vi "LVFPGA Tx.vi"(0 "device name":string="RIO0", 1 "Enabled Channels":string(combo)="0", 5 "IQ rate":dbl=10000000.0 caption="IQ Rate" format="%#.3pS/s", 7 "number of samples":i64=16384 caption="Number of Samples", 9 "run duration":dbl=5.0 format="%#_13g", 11 "error in":errorcluster) -> (6 "coerced IQ rate":dbl format="%#_6p", 8 "underflow":bool, 10 "overflow":bool, 15 "error out":errorcluster)   [LabVIEW 2015]
doc: "This template is for the Simple NI-USRP Streaming design, a design that shows the basics of streaming data to an NI USRP-294x/295x device. Refer to the block diagram for more information about how to use this template."
uses:
  SubVIs/niusrprios Write Tx Data (I16 multi).vi
  SubVIs/niusrprios Start Trigger.ctl
  SubVIs/niusrprios Configure Signal (Level).vi
  SubVIs/niusrprios Generate Waveform (Interleaved).vi
panel:
  in  "which bitfile":string(combo)="Time"
  in  "Reference Frequency Source":string(combo)="Internal"
  out "generating":bool caption="Generating"
  in  "number of samples is finite":bool
  in  "stop":bool
  # "Tx Streaming"
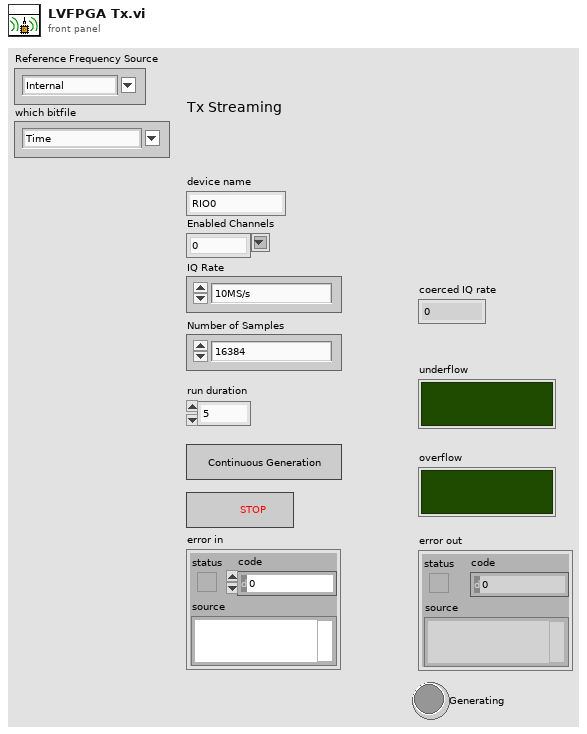
[diagram p1: front panel]
types:
  T1 = typedef "niusrprios Start Trigger.ctl" = enum8{"Software", "Digital Edge", "Rx Start Trigger", "Tx Start Trigger", "Immediate", "Future Time Event"}
  T2 = cluster{"antenna":string, "frequency":dbl, "lo frequency":dbl, "level":dbl}
  T3 = cluster{"channel enable":bool, "channel configuration":cluster{"antenna":string, "frequency":dbl, "lo frequency":dbl, "level":dbl}}
  T4 = cluster{"antenna":string, "frequency":dbl, "lo frequency":dbl, "level":dbl}[]
  T5 = typedef "niUsrpRio Config v1 Host.lvlib/niUsrpRio Session.ctl" = cluster{"FPGA Interface":refnum<k20>, "RIO Interface Number":u32, "Data Clock Rate":u32, "FPGA Data Clock Rate":u32, "Global Settings Register Bus":T6, "Radio 0 Settings Register Bus":T6, "Radio 1 Settings Register Bus":T6, "Radio Settings Bus Semaphore":T7, "DB Queues":T8[], "Characterization Data Valid?":bool, "EEPROM Header":T9, "Device Data Header":T10, "EEPROM Characterization Header":T11, "Characterization Data":T12[], "FPGA Current Version":u32, "FPGA Oldest Compatible Version":u32, "Fixed Logic Current Version":u32, "Fixed Logic Oldest Compatible Version":u32, "FPGA Radio Settings Bus Current Version":u32, "FPGA Radio Settings Bus Oldest Compatible Version":u32, "FPGA Board Config Current Version":u32, "FPGA Board Config Oldest Compatible Version":u32, "Daughterboard Clock Rate":u32}
  T6 = typedef "niInstr Register Bus v0 Host.lvlib/Register Bus Session.ctl" = refnum<queue>
  T7 = typedef "Semaphore RefNum" = refnum<k1>
  T8 = typedef "niUsrpRio Config v1 Host.lvlib/DB Queue Reference.ctl" = refnum<queue>
  T9 = typedef "niUsrpRio Config v1 Host.lvlib/EEPROM Header.ctl" = cluster{"Checksum":u32, "Product Code":u16, "Hardware Current Version":u16, "Hardware Oldest Compatible Version":u16, "EEPROM Map Current Version":u16, "EEPROM Map Oldest Compatible Version":u16, "User Password":string, "Pointer to Factory Header":u32, "Pointer to User Header":u32, "Recommended Interval":u16, "Number of Reserved Bytes":i32, "Number of Daughterboards":u8, "Daughterboard IDs":u16[], "Daughterboard Serial Numbers":string[]}
  T10 = typedef "niUsrpRio Config v1 Host.lvlib/EEPROM Device Data Header.ctl" = cluster{"Checksum":u32, "Number of Channels":u8, "Number of Gain Settings":u16[], "Pointer to Characterization Data":u32[], "Number of Reserved Bytes":i32, "Number of Frequencies":u16[]}
  T11 = typedef "niUsrpRio Config v1 Host.lvlib/EEPROM Characterization Header.ctl" = cluster{"Checksum":u32, "Date":timestamp, "Temperature":sgl, "Misc. Info":string, "Pointer to Device Data Header":u32, "Number of Reserved Bytes":i32}
  T12 = typedef "niUsrpRio Config v1 Host.lvlib/Characterization Data.ctl" = cluster{"Gains[dB]":dbl[], "Frequencies [Hz]":dbl[], "IQ Imbalance Table":T13[], "Measured Gains[dB]":dbl[][]}
  T13 = typedef "niUsrpRio Config v1 Host.lvlib/IQ Imbalance.ctl" = cluster{"Gain Imbalance [linear]":dbl, "Phase Imbalance [radians]":dbl, "Offset":cdb}
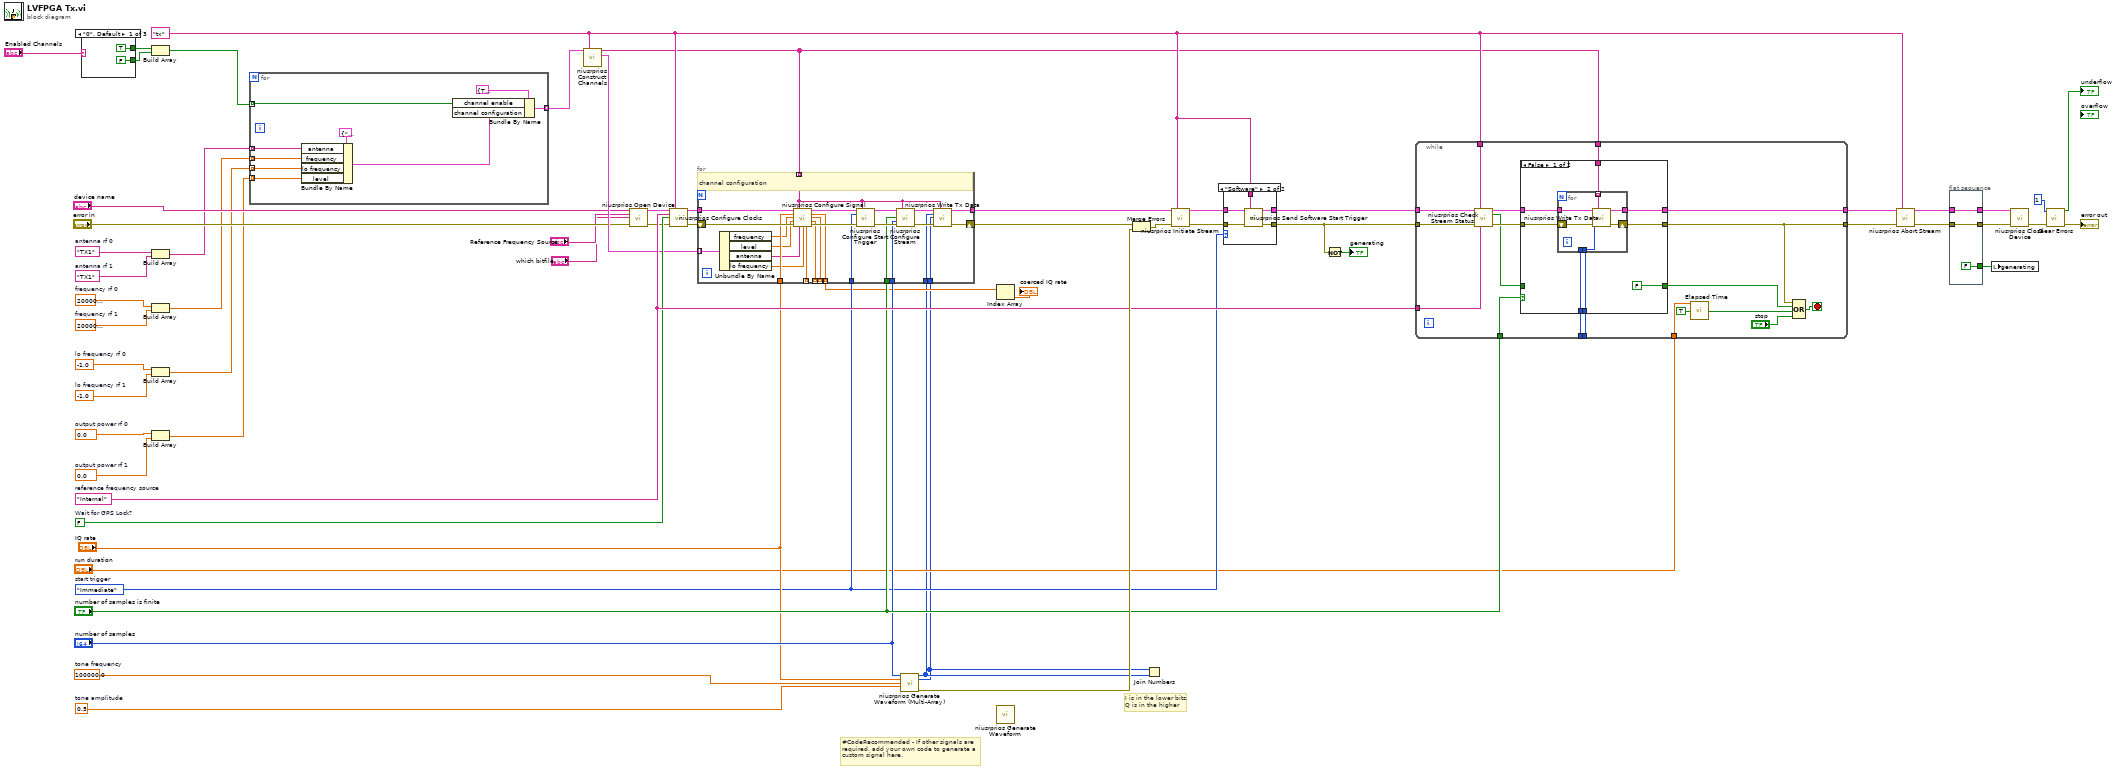
[diagram p0: block diagram]
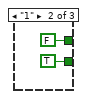
[diagram p2: hidden frame]
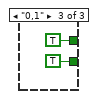
[diagram p3: hidden frame]
diagram:
  w48 = 100000.0  # tone frequency
  w39 = niusrprios_Start_Trigger."Immediate"  # start trigger
  w62 = "Internal"  # reference frequency source
  w53 = 0.0  # output power rf 1
  w52 = 0.0  # output power rf 0
  w54 = -1.0  # lo frequency rf 1
  w55 = -1.0  # lo frequency rf 0
  w56 = 2000000000.0  # frequency rf 1
  w57 = 2000000000.0  # frequency rf 0
  w59 = "TX1"  # antenna rf 1
  w58 = "TX1"  # antenna rf 0
  w40 = FALSE  # Wait for GPS Lock?
  w47 = 0.5  # tone amplitude
  w35 = "tx" ("scope")
  # "I is in the lower bits,\nQ is in the higher"
  # "#CodeRecommended - If other signals are required, add your own code to generate a custom signal here."
  n1 = case shown="\"0\", Default" "Enabled Channels" {
    tunnel: [TRUE FALSE TRUE] -> w21
    tunnel: [FALSE TRUE TRUE] -> w20
    frame "0", Default {
    }
    frame "1" {
    }
    frame "0,1" {
    }
  }
  n2 = Build Array(w21, w20) -> (w12:bool[])
  n3 = Build Array(w58, w59) -> (w11:string[])
  n4 = Build Array(w57, w56) -> (w10:dbl[])
  n5 = Build Array(w55, w54) -> (w9:dbl[])
  n6 = Build Array(w52, w53) -> (w8:dbl[])
  n7 = for {
    tunnel: w12 -> [w77] mode=indexing
    tunnel: w11 -> [w75] mode=indexing
    tunnel: w10 -> [w74] mode=indexing
    tunnel: w9 -> [w73] mode=indexing
    tunnel: w8 -> [w72] mode=indexing
    tunnel: [w70] -> w7 mode=indexing
    n8 = Bundle By Name(cluster=T2 {"antenna"="", "frequency"=0.0, "lo frequency"=0.0, "level"=0.0} ("channel configuration"), "antenna"=w75, "frequency"=w74, "lo frequency"=w73, "level"=w72) -> (w71:T2)
    n9 = Bundle By Name(cluster=T3 {"channel enable"=TRUE, "channel configuration"={"antenna"="RX1", "frequency"=2000000000.0, "lo frequency"=-1.0, "level"=0.0}} ("channel configuration"), "channel enable"=w77, "channel configuration"=w71) -> (w70:T3)
  }
  n10 = call "niusrprios Construct Channels.vi"("channel configurations"=w7, "scope"=w35) -> ("enabled channels"=w34:string[], "enabled channel configurations"=w33:T4)  [unwired: 12 in]
  n11 = call "niusrprios Open Device.vi"("USRP RIO device"="device name", "Reference Frequency Source"="Reference Frequency Source", "which bitfile"="which bitfile", "error in"="error in") -> ("niUsrpRio Session (out)"=w32:T5, "error out"=w31:errorcluster)  [unwired: 10 in]
  n12 = call "niusrprios Configure Clocks.vi"("niUsrpRio Session"=w32, "scope"=w35, "Reference Frequency Source"=w62, "GPSDO Power Enable"=w40, "error in"=w31) -> ("niUsrpRio Session (out)"=w29:T5, "error out"=w30:errorcluster)  [unwired: 9 in]
  n13 = call "niusrprios Generate Waveform (Multi-Array).vi"("number of samples"="number of samples", "sample rate"="IQ rate", "tone frequency"=w48, "amplitude"=w47) -> ("I"=w4:i16[], "Q"=w3:i16[], "error out"=w63:errorcluster)  [unwired: 8 in, 1 out]
  n14 = for {
    tunnel: [w87] -> _ mode=indexing
    tunnel: [w92] -> w27
    tunnel: w39 -> [w102]
    tunnel: "number of samples" -> [w97]
    tunnel: "number of samples is finite" -> [w96]
    shift-right: [w94] -> w26
    shift-left: w30 -> [w98]
    tunnel: w34 -> [w91] mode=indexing
    tunnel: "IQ rate" -> [w95]
    tunnel: w3 -> [w90]
    tunnel: w4 -> [w89]
    tunnel: w29 -> [w88]
    tunnel: [w86] -> _ mode=indexing
    tunnel: [w85] -> _ mode=indexing
    tunnel: [w84] -> w24 mode=indexing
    tunnel: w33 -> [w83] mode=indexing
    # "channel configuration"
    n15 = Unbundle By Name(w83) -> ("frequency"=w82:dbl, "level"=w81:dbl, "antenna"=w80:string, "lo frequency"=w79:dbl)
    n16 = call-poly "niusrprios Configure Signal.vi"("niUsrpRio Session"=w88, "scope"=w91, "sample rate [S/s]"=w95, "frequency [Hz]"=w82, "level [dBm]"=w81, "error in"=w98, "Active Antenna"=w80, "LO frequency [Hz]"=w79) -> ("niUsrpRio Session (out)"=w100:T5, "coerced sample rate [S/s]"=w84:dbl, "coerced frequency [Hz]"=w85:dbl, "coerced level [dBm]"=w86:dbl, "coerced LO frequency [Hz]"=w87:dbl, "error out"=w104:errorcluster)  [unwired: 1 in, 1 out]
    n17 = call "niusrprios Configure Start Trigger.vi"("niUsrpRio Session"=w100, "scope"=w91, "start trigger"=w102, "error in"=w104) -> ("niUsrpRio Session (out)"=w99:T5, "error out"=w101:errorcluster)  [unwired: 10 in]
    n18 = call "niusrprios Configure Stream.vi"("niUsrpRio Session"=w99, "scope"=w91, "number of samples is finite"=w96, "number of samples"=w97, "error in"=w101) -> ("niUsrpRio Session (out)"=w93:T5, "error out"=w103:errorcluster)  [unwired: 9 in]
    n19 = call-poly "niusrprios Write Tx Data.vi"("niUsrpRio Session"=w93, "scope"=w91, "I"=w89, "Q"=w90, "error in"=w103) -> ("niUsrpRio Session (out)"=w92:T5, "error out"=w94:errorcluster)  [unwired: 9 in]
  }
  n20 = Index Array(array=w24) -> (element=→"coerced IQ rate":dbl)  [unwired: 1 in]
  n21 = call-poly "niusrprios Generate Waveform.vi"() -> ()  [unwired: 13 in, 3 out]
  n22 = Merge Errors(w26, w63) -> (w25:errorcluster)
  n23 = Join Numbers(hi=w3, lo=w4) -> ()  [unwired: 1 out]
  n24 = call "niusrprios Initiate Stream.vi"("niUsrpRio Session"=w27, "scope"=w35, "error in"=w25) -> ("niUsrpRio Session (out)"=w36:T5, "error out"=w37:errorcluster)  [unwired: 11 in]
  n25 = case shown="\"Software\"" w39 {
    tunnel: w37 -> [w106 w111]
    tunnel: [w106 w110] -> w38
    tunnel: w36 -> [w105 w109]
    tunnel: w35 -> [_ w108]
    tunnel: [w105 w107] -> w28
    frame Default {
    }
    frame "Software" {
      n26 = call "niusrprios Send Software Start Trigger.vi"("niUsrpRio Session"=w109, "scope"=w108, "error in"=w111) -> ("niUsrpRio Session (out)"=w107:T5, "error out"=w110:errorcluster)  [unwired: 11 in]
    }
  }
  n27 = Not(x=w38) -> (.not. x?=→"generating":bool)
  n28 = while {
    tunnel: [w128] -> w61
    tunnel: [w127] -> w60
    tunnel: "number of samples is finite" -> [w118]
    tunnel: w34 -> [w126]
    tunnel: [w125] -> w1
    tunnel: [w124] -> w2
    tunnel: w38 -> [w122]
    tunnel: w28 -> [w123]
    tunnel: w35 -> [w116]
    tunnel: w62 -> [w115]
    tunnel: "run duration" -> [w112]
    stop <- w130 stop-if-true
    # "Acquire and Fetch a waveform"
    n29 = call "niusrprios Check Stream Status.vi"("niUsrpRio Session"=w123, "scope"=w116, "error in"=w122, "reference frequency source"=w115) -> ("niUsrpRio Session (out)"=w121:T5, "done"=w119:bool, "error out"=w120:errorcluster)  [unwired: 9 in]
    n30 = case shown="False" w118 {
      tunnel: [w138 w147] -> w128
      tunnel: [w137 w148] -> w127
      tunnel: w126 -> [w136 _]
      tunnel: w125 -> [w135 _]
      tunnel: w124 -> [w134 _]
      tunnel: w121 -> [w133 w147]
      tunnel: w120 -> [w132 w148]
      tunnel: [FALSE w146] -> w117
      tunnel: w119 -> [_ w146]
      frame False {
        n31 = for {
          shift-right: [w144] -> w137
          shift-left: w132 -> [w145]
          tunnel: w136 -> [w142] mode=indexing
          tunnel: w133 -> [w143]
          tunnel: [w141] -> w138
          tunnel: w134 -> [w140]
          tunnel: w135 -> [w139]
          n32 = call-poly "niusrprios Write Tx Data.vi"("niUsrpRio Session"=w143, "scope"=w142, "I"=w139, "Q"=w140, "error in"=w145) -> ("niUsrpRio Session (out)"=w141:T5, "error out"=w144:errorcluster)  [unwired: 9 in]
        }
      }
      frame True {
      }
    }
    n33 = call "Elapsed Time"("Time Target (s)"=w112, "Auto Reset"=TRUE) -> ("Time has Elapsed"=w113:bool)  [unwired: 10 in, 7 out]
    n34 = Compound Arithmetic op=OR(w127, w117, w113, "stop") -> (w130:bool)
  }
  n35 = call "niusrprios Abort Stream.vi"("niUsrpRio Session"=w61, "scope"=w35, "error in"=w60) -> ("niUsrpRio Session (out)"=w45:T5, "error out"=w46:errorcluster)  [unwired: 11 in]
  n36 = flat-sequence {
    tunnel: [w151] -> w44
    tunnel: w45 -> [w151]
    tunnel: [w150] -> w43
    tunnel: w46 -> [w150]
    tunnel: [FALSE ("Generating")] -> w42
    frame #0 {
    }
  }
  n37 = local write "generating"(w42) -> ()
  n38 = call "niusrprios Close Device.vi"("niUsrpRio Session"=w44, "error in"=w43) -> ("error out"=w18:errorcluster)  [unwired: 13 in]
  n39 = call <vilib>:"Clear Errors.vi"("error in (no error)"=w18, "specific error code to clear (0: all)"=1) -> ("error out"=→"error out":errorcluster, "specific error cleared?"=→"underflow":bool)  [unwired: 4 in]
